vi "UnFlatten Test Parameters.vi"(4 "error in (no error)":errorcluster, 7 "Flattened Test Parameters with Version (\"\")":string) -> (0 "error out":errorcluster, 2 "Test Version":string, 3 "Flat Test Parameters":string)   [LabVIEW 2011]
uses:
  Flat Report Parameters Cluster.ctl
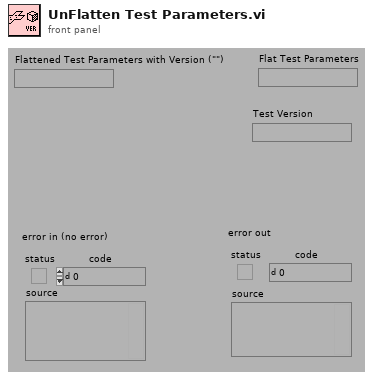
[diagram p1: front panel]
types:
  T1 = typedef "Flat Report Parameters Cluster.ctl" = cluster{"Flattened Test Version":string, "Flattened Test Parameters":string}
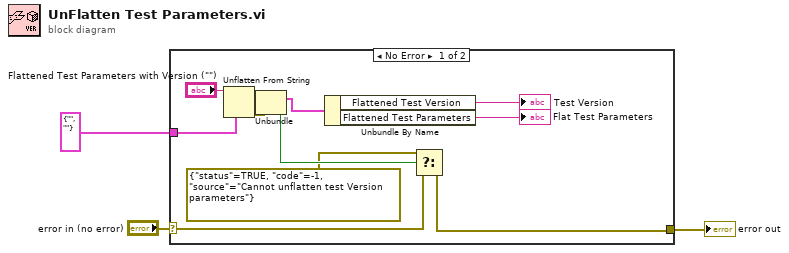
[diagram p0: block diagram]
diagram:
  n1 = case shown="No Error" "error in (no error)" {
    selector: "error in (no error)" -> [w7 w14]
    tunnel: [w8 w14] -> w3
    tunnel: T1 {"Flattened Test Version"="", "Flattened Test Parameters"=""} ("Test Report Parameters") -> [w5 _]
    frame No Error {
      n2 = Unflatten From String(type=w5, binary string="Flattened Test Parameters with Version (\"\")") -> (value=w12:T1, error out=w4:errorcluster)  [unwired: 1 in, 3 out]
      n3 = Unbundle(w4) -> ("status"=w10:bool)  [unwired: 2 out]
      n4 = Unbundle By Name(w12) -> ("Flattened Test Version"=→"Test Version":string, "Flattened Test Parameters"=→"Flat Test Parameters":string)
      n5 = Select(t=errorcluster {"status"=TRUE, "code"=-1, "source"="Cannot unflatten test Version parameters"}, s=w10, f=w7) -> (s? t:f=w8:errorcluster)
    }
    frame Error {
    }
  }
  "error out" <- w3
